vi "Frame create.vi"(7 "Command":string, 8 "error in (no error)":errorcluster, 11 "ISO 14443 A DOWN in":refnum<class "ISO 14443 A DOWN.lvclass">) -> (0 "error out":errorcluster, 3 "ISO 14443 A DOWN out":refnum<class "ISO 14443 A DOWN.lvclass">)   [LabVIEW 2019, in "ISO 14443 A DOWN.lvclass"]
uses:
  ISO 14443 A DOWN.lvclass
  TypeDef/Store.ctl
  ISO 14443 A DOWN.lvclass/ISO 14443 A DOWN.ctl
  RFID system.lvclass
panel:
  in  "WUPA":u8[](array[numeric])=[38] format="%x"
  # "REQA"
  # "WUPA"
  # "0"
  # "1"
  # "1"
  # "0"
  # "0"
  # "1"
  # "0"
  # "0"
  # "1"
  # "0"
  # "0"
  # "1"
  # "0"
  # "1"
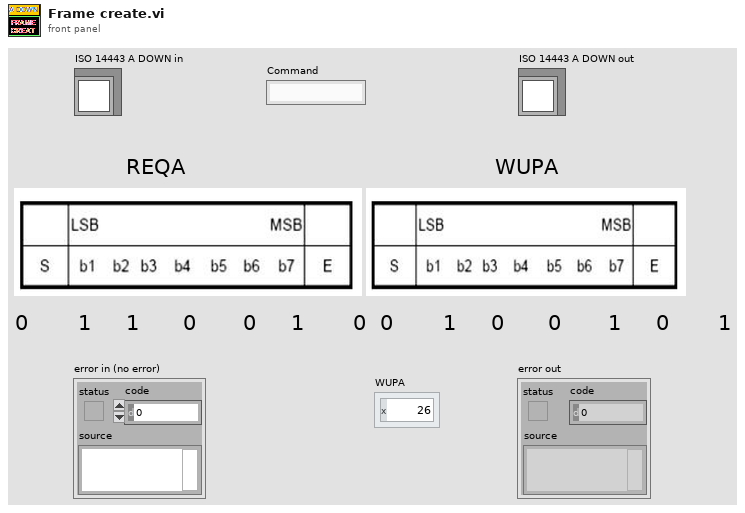
[diagram p1: front panel]
types:
  T1 = typedef "Store.ctl" = enum16{"envelope", "noise", "demSubCar", "CH_frame", "Decode", "demodulate", "in", "out", "sum", "subCarrier", "frame", "command", "encode", "modulate", "encode_UP", "modulate_up", "demod_up", "envelop_up", "sum_up", "out_up", "in_up"}
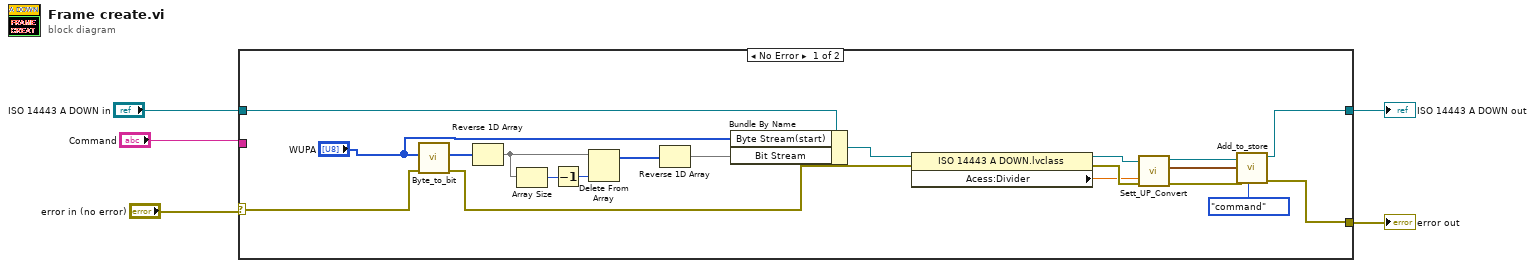
[diagram p0: block diagram]
diagram:
  n1 = case shown="No Error" "error in (no error)" {
    selector: "error in (no error)" -> [w22 w26]
    tunnel: "ISO 14443 A DOWN in" -> [w21 w27]
    tunnel: [w17 w27] -> w3
    tunnel: "Command" -> [_ _]
    tunnel: [w15 w26] -> w2
    frame No Error {
      n2 = call "Byte_to_bit.vi"("Error In"=w22, "Array of byte"="WUPA") -> ("Error Out"=w12:errorcluster, "Arrray of bit"=w25:u8[])  [unwired: 5 in, 1 out]
      n3 = Reverse 1D Array(array=w25) -> (reversed array=w9:u8[])
      n4 = Array Size(array=w9) -> (size(s)=w24:i32)
      n5 = Decrement(x=w24) -> (x-1=w23:i32)
      n6 = Delete From Array(array=w9, index=w23) -> (array with subset deleted=w7:u8[])  [unwired: 1 in, 1 out]
      n7 = Reverse 1D Array(array=w7) -> (reversed array=w6:u8[])
      n8 = Bundle By Name(cluster=w21, "Byte Stream(start)"="WUPA", "Bit Stream"=w6) -> (w20:refnum<class "ISO 14443 A DOWN.lvclass">)
      n9 = property class="ISO 14443 A DOWN.lvclass"(reference=w20, error in=w12) -> (reference out=w13:refnum<class "ISO 14443 A DOWN.lvclass">, error out=w11:errorcluster, "Acess:Divider"=w10:dbl)
      n10 = call-dynamic "Sett_UP_Convert.vi"("error in (no error)"=w11, "Divider(1)"=w10, "ISO 14443 A DOWN in"=w13) -> ("error out"=w16:errorcluster, "Waveform"=w19:waveform(dbl), "ISO 14443 A DOWN out"=w18:refnum<class "ISO 14443 A DOWN.lvclass">)  [unwired: 6 in]
      n11 = call "Add_to_store.vi"("Store"=Store."command", "error in (no error)"=w16, "Waveform"=w19, "RFID system in"=w18) -> ("error out"=w15:errorcluster, "RFID system out"=w17:refnum<class "ISO 14443 A DOWN.lvclass">)  [unwired: 6 in]
    }
    frame Error {
    }
  }
  "error out" <- w2
  "ISO 14443 A DOWN out" <- w3
